vi "Count non NaN values.vi"(5 "array in":sgl[](array[numeric])=[35.0, nan, 0.0]) -> (1 "count":i32=2)   [LabVIEW 2009]
doc: "Counts number of non NaN values in array"
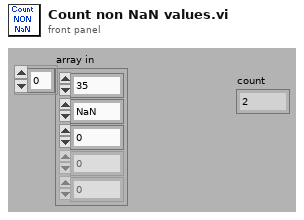
[diagram p1: front panel]
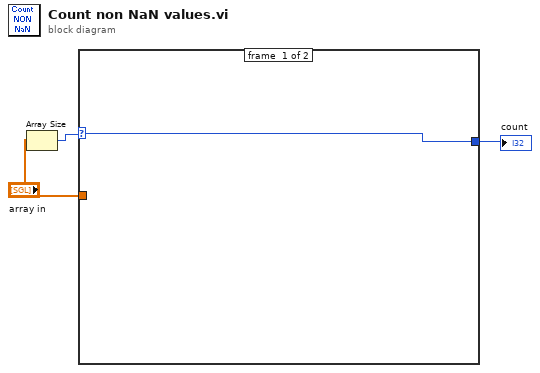
[diagram p0: block diagram]
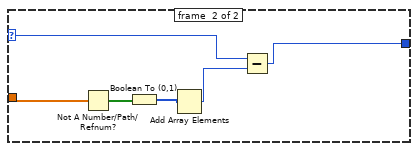
[diagram p2: hidden frame]
diagram:
  n1 = Array Size(array="array in") -> (size(s)=w2:i32)
  n2 = case shown="1, Default" w2 {
    selector: w2 -> [w4 w7]
    tunnel: "array in" -> [_ w10]
    tunnel: [w4 w5] -> w1
    frame #0 {
    }
    frame #1 {
      n3 = Not A Number/Path/Refnum?(number/path/refnum=w10) -> (NaN/Path/Refnum?=w9:bool[])
      n4 = Boolean To (0,1)(Boolean=w9) -> (0, 1=w8:i16[])
      n5 = Add Array Elements(numeric array=w8) -> (sum=w6:i16)
      n6 = Subtract(x=w7, y=w6) -> (x-y=w5:i32)
    }
  }
  "count" <- w1
